vi "ProgressBar-Call fileGen progress window.vi"(8 "error in (no error)":errorcluster, 11 "Z-stack queue cluster":T1={"Imaging Protocol"=enum."Live Imaging", "Number of Trials"=0, "Frame Size"=512, "# Averaged frames"=0, "Dwell time (us)"=0.0, "Index of Z-plane"=0, "Timelapse?"=FALSE, "Logging process is active"=FALSE, "Speed logging enabled"=FALSE, "tdms file ref"=refnum, "path"=path "", "Trial Number"=0, "Expected # points acquired"=FALSE, "Manually stopped"=FALSE, "Last trial"=FALSE, "Ch0 data"=[], "Ch1 data"=[], "Image Time"=[], "Continuous Time"=[], "Points acquired"={"Ch0 last trial"=0, "Ch1 last trial"=0, "All trials"=0}, "HW Timings File"=refnum} {"Frame Size" items=["100X100"=100, "128X128"=128, "200X200"=200, "256X256"=256, "512X512"=512, "1024x1024"=1024, "2048x2048"=2048]; "Dwell time (us)" format="%#.6g"}) -> (0 "error out":errorcluster)   [LabVIEW 2017]
uses:
  Typedefs/Logging queue element.ctl
  Typedefs/Imaging Protocols enum.ctl
  Typedefs/Frame Size.ctl
  Typedefs/Acquired points count.ctl
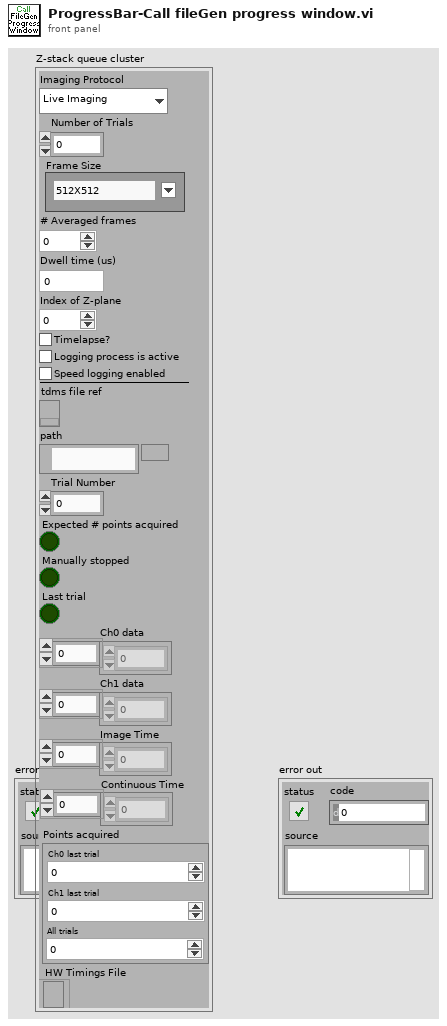
[diagram p1: front panel]
types:
  T1 = typedef "Logging queue element.ctl" = cluster{"Imaging Protocol":T2, "Number of Trials":u16, "Frame Size":T3, "# Averaged frames":u16, "Dwell time (us)":dbl, "Index of Z-plane":i32, "Timelapse?":bool, "Logging process is active":bool, "Speed logging enabled":bool, "tdms file ref":refnum<k34>, "path":path, "Trial Number":i32, "Expected # points acquired":bool, "Manually stopped":bool, "Last trial":bool, "Ch0 data":u32[], "Ch1 data":u32[], "Image Time":u64[], "Continuous Time":u64[], "Points acquired":T4, "HW Timings File":refnum<file>}
  T2 = typedef "Imaging Protocols enum.ctl" = enum16{"AOL Z-Stack", "Motor Z Stack", "Functional Acquisition", "Single Plane Acquisition", "Volume Acquisition", "Live Imaging", "Live Plane Imaging", "Live Volume Imaging"}
  T3 = typedef "Frame Size.ctl" = u16
  T4 = typedef "Acquired points count.ctl" = cluster{"Ch0 last trial":u64, "Ch1 last trial":u64, "All trials":u64}
  T5 = typedef "Progress bar window values input cluster.ctl" = cluster{"Total":i32, "Current":i32, "Message in":string, "Sender":enum16{"Acquisition", "Logging", "File gen"}}
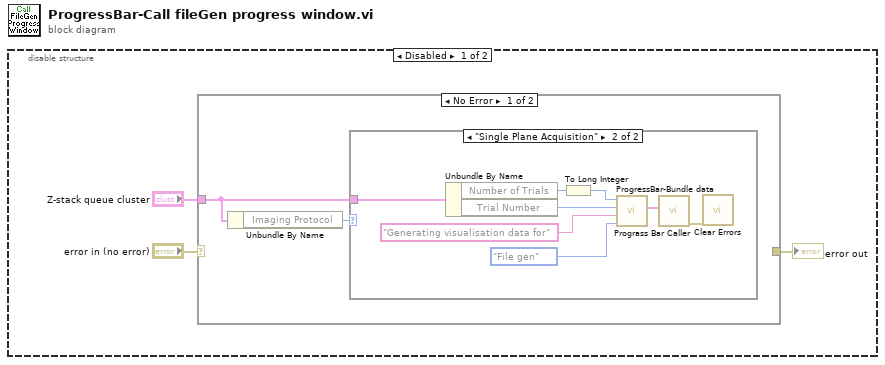
[diagram p0: block diagram]
diagram:
  n1 = disable-structure shown="Disabled" {
    frame Disabled {
      n2 = case shown="No Error" "error in (no error)" {
        selector: "error in (no error)" -> [_ w14]
        tunnel: "Z-stack queue cluster" -> [w5 _]
        tunnel: [_ w14] -> w1
        frame No Error {
          n3 = Unbundle By Name(w5) -> ("Imaging Protocol"=w4:T2)
          n4 = case shown="\"Single Plane Acquisition\"" w4 {
            tunnel: w5 -> [_ w12]
            frame Default {
            }
            frame "Single Plane Acquisition" {
              n5 = Unbundle By Name(w12) -> ("Number of Trials"=w13:u16, "Trial Number"=w11:i32)
              n6 = To Long Integer(number=w13) -> (32bit integer=w7:i32)
              n7 = call "ProgressBar-Bundle data.vi"("Sender"=enum16{"Acquisition", "Logging", "File gen"}."File gen", "Message in"="Generating visualisation data for" ("string"), "Current"=w11, "Total"=w7) -> ("Progress bar window values input"=w10:T5)  [unwired: 7 in]
              n8 = call "Prograss Bar Caller.vi"("Progress bar window values input"=w10) -> ("error out"=w8:errorcluster)  [unwired: 10 in]
              n9 = call <vilib>:"Clear Errors.vi"("error in (no error)"=w8) -> ()  [unwired: 5 in, 2 out]
            }
          }
        }
        frame Error {
        }
      }
      "error out" <- w1
    }
    frame Enabled {
    }
  }
